vi "Keithley 2600 Series Merge NEW.vi"() -> ()   [LabVIEW 2017]
doc: "This example shows how to create, run a script and query the script output data."
uses:
  <vilib>/Utility/file.llb/Write Delimited Spreadsheet (DBL).vi
  <instrlib>/Keithley 2600 Series/Keithley 2600 Series.lvlib
panel:
  out "Sweep":i32
  in  "Yes":bool
  out "First Sweep 2":bool
  in  "No":bool
  out "Graph 2":cluster{"Y":dbl[], "Y":dbl[]}[](graph)
  out "output array":string[][](array[string])
  out "Seconds":i32
  out "Minutes":i32
  out "Hours":i32
  in  "Stop Button":bool
  in  "Number of Sweeps":dbl=10.0 min=1.0 max=1000.0 step=1.0
  in  "Aperture State (Channel B)":u16(ring) items=["Always OFF", "Always ON", "ON During Sweep OFF Otherwise", "OFF During Sweep ON Otherwise"]
  in  "Inter Sweep Delay(s)":dbl=0.1 min=0.1 max=3600.0
  out "Working Folder":path
  in  "Folder Name":string="Raw Measurement"
  in  "Sweep Setting (Channel A)":T1={"Start Voltage(V)"=0.0, "Stop Voltage(V)"=0.0, "Number of Points"=10.0, "Settling Time(s)"=0.1, "Current Limit(A)"=0.1} {"Current Limit(A)" min=0.1 max=1.5; "Settling Time(s)" min=0.1 max=60.0; "Number of Points" min=10.0 max=10000.0 step=1.0; "Stop Voltage(V)" min=0.0 max=200.0; "Start Voltage(V)" min=0.0 max=200.0}
  in  "USB COM Port":refnum<visa-resource-name>
  # "Time Remaining"
  # ":"
  # ":"
  # "2634B can output up to 20.2 V at 1.5 A,\n or 202 V at 100 mA current limit."
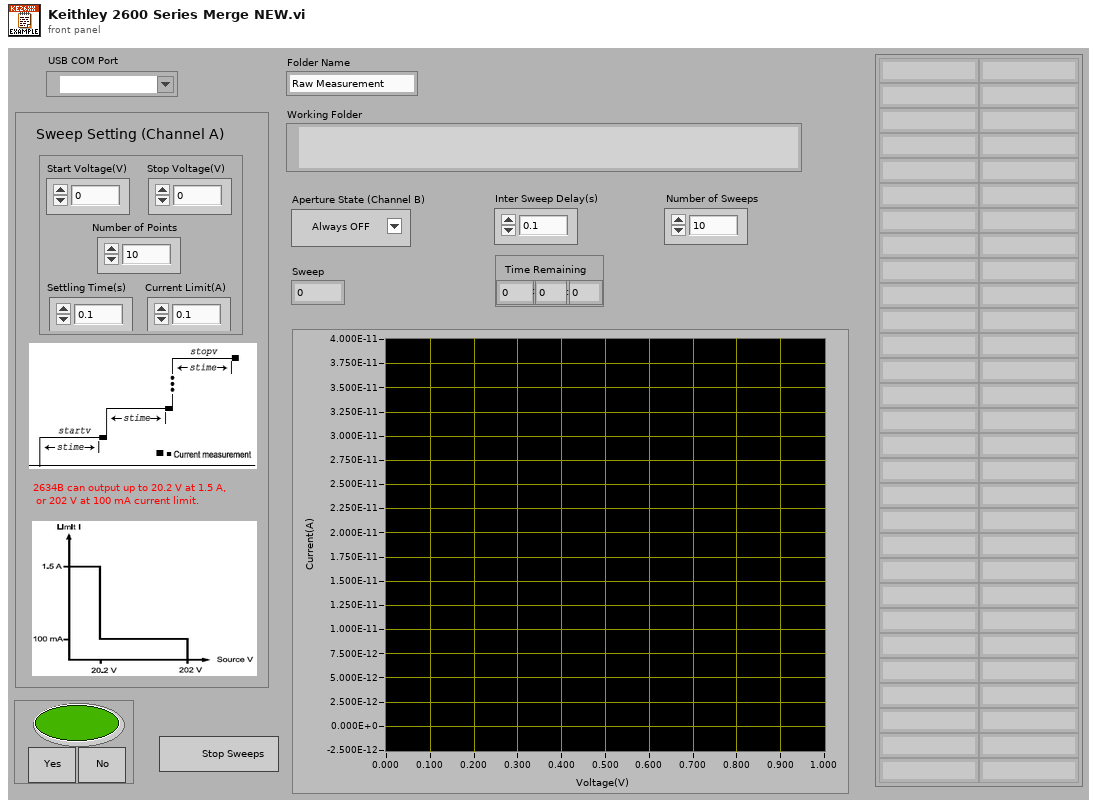
[diagram p1: front panel]
types:
  T1 = cluster{"Start Voltage(V)":dbl, "Stop Voltage(V)":dbl, "Number of Points":dbl, "Settling Time(s)":dbl, "Current Limit(A)":dbl}
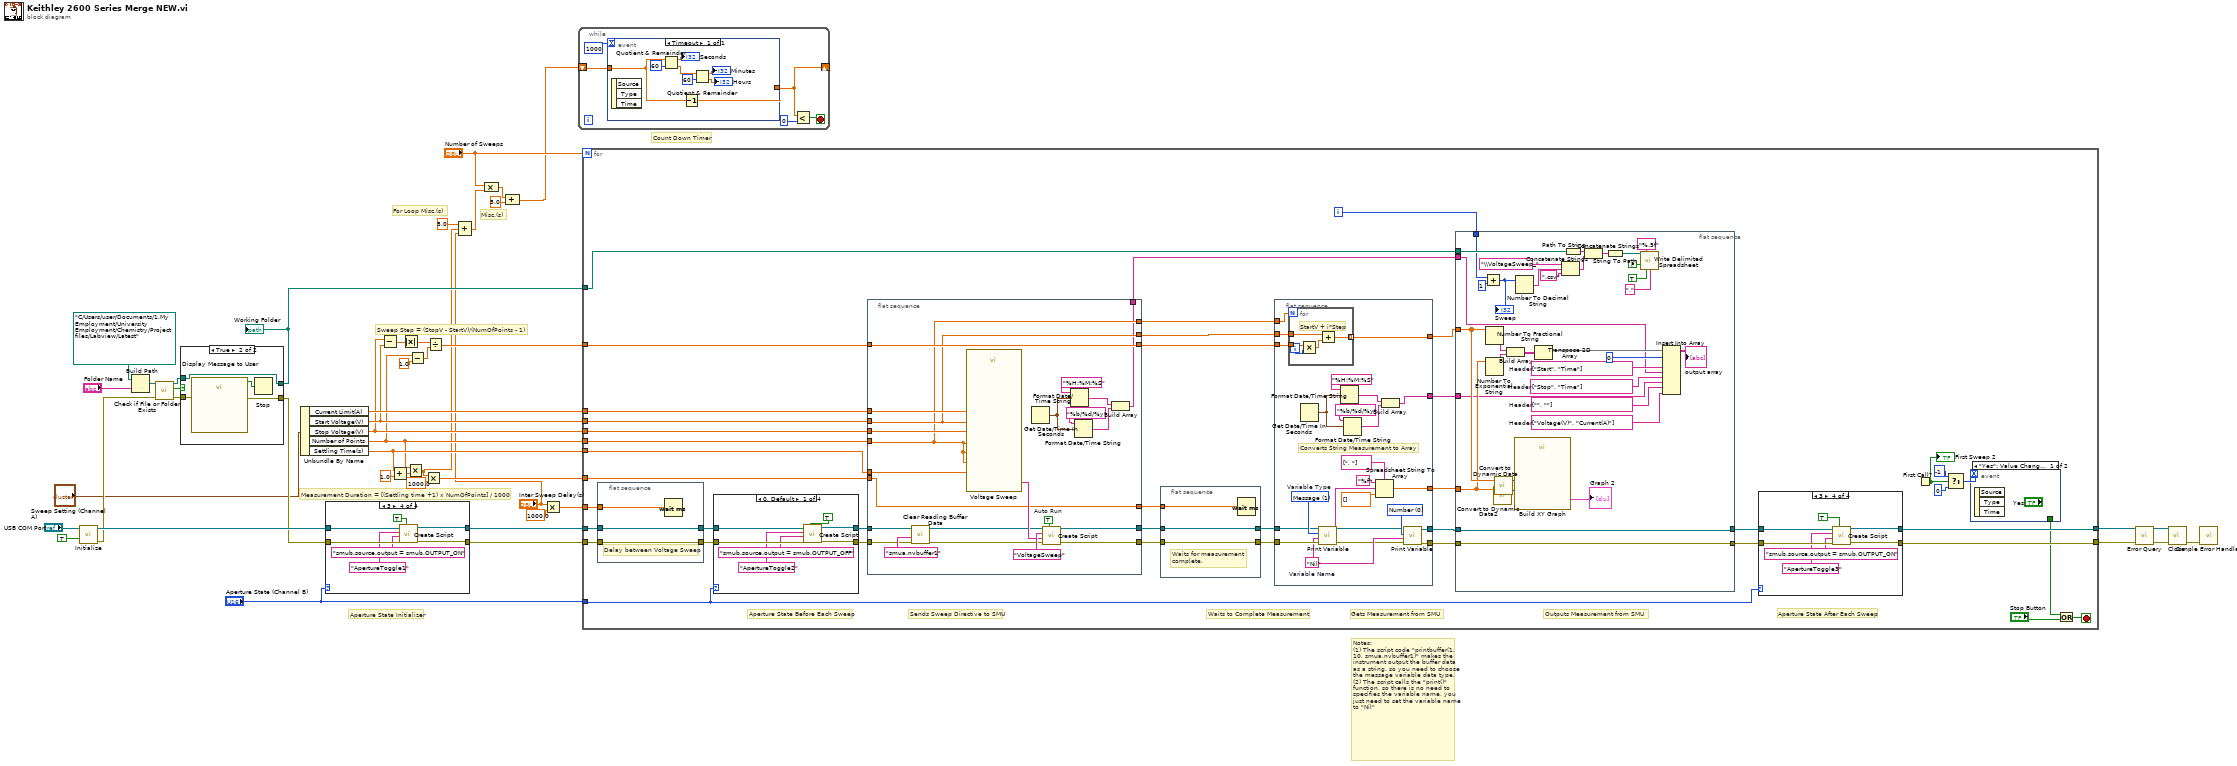
[diagram p0: block diagram]
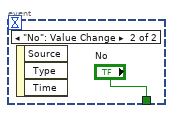
[diagram p2: hidden frame]
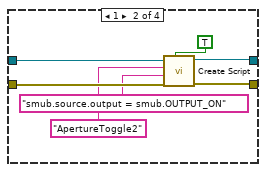
[diagram p3: hidden frame]
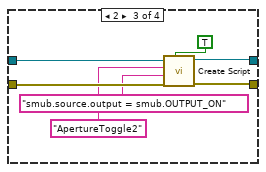
[diagram p4: hidden frame]
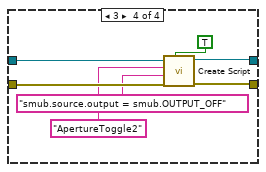
[diagram p5: hidden frame]
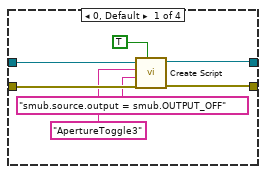
[diagram p6: hidden frame]
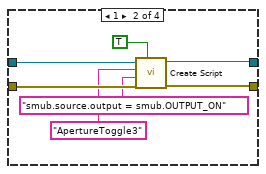
[diagram p7: hidden frame]
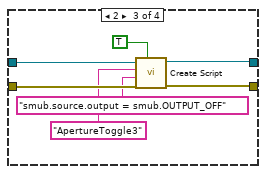
[diagram p8: hidden frame]
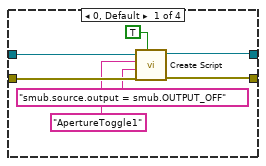
[diagram p9: hidden frame]
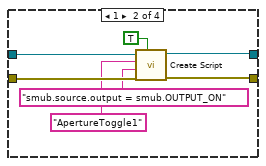
[diagram p10: hidden frame]
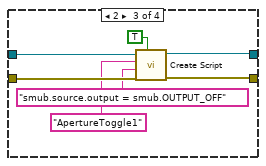
[diagram p11: hidden frame]
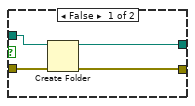
[diagram p12: hidden frame]
diagram:
  # "Count Down Timer"
  # "Misc.(s)"
  # "For Loop Misc.(s)"
  # "Sweep Step = (StopV - StartV)/(NumOfPoints - 1)"
  # "Measurement Duration = [(Settling time +1) x NumOfPoints] / 1000"
  # "Aperture State Initializer"
  # "Notes: \n(1) The script code \"printbuffer(1, 10, smua.nvbuffer1)\" makes the instrument output the buffer data as a string, so you need to choose the message variable data type.\n(2) The script calls the \"print()\" function, so there is no need to specifies the variable name, you just need to set the variable name to \"Nil\""
  n1 = call <instrlib>:"Initialize.vi"("Reset (True)"=TRUE, "VISA resource name"="USB COM Port") -> ("error out"=w28:errorcluster, "VISA resource name out"=w29:refnum<visa-resource-name>)  [unwired: 8 in]
  n2 = Build Path(base path=path "C:/Users/user/Documents/1.My Employment/University Employment/Chemistry/Project files/Labview/Latest" ("Working Directory"), name or relative path="Folder Name") -> (appended path=w38:path)
  n3 = call <vilib>:"Check if File or Folder Exists.vi"("error in (no error)"=w28, "path"=w38) -> ("error out"=w35:errorcluster, "file or folder exists?"=w37:bool, "dup path"=w36:path)  [unwired: 7 in]
  n4 = case shown="True" w37 {
    tunnel: [w48 w51] -> w34
    tunnel: w36 -> [w49 w51]
    tunnel: w35 -> [w47 w53]
    tunnel: [w46 w50] -> w27
    frame False {
      n5 = Create Folder(path (use dialog)=w49, error in=w47) -> (created path=w48:path, error out=w46:errorcluster)  [unwired: 1 in, 1 out]
    }
    frame True {
      n6 = call "Display Message to User"("error in (no error)"=w53) -> ("error out"=w50:errorcluster, "OK"=w52:bool)  [unwired: 9 in]
      n7 = Stop(stop? (T)=w52) -> ()
    }
  }
  "Working Folder" <- w34
  n8 = Unbundle By Name("Sweep Setting (Channel A)") -> ("Current Limit(A)"=w24:dbl, "Start Voltage(V)"=w13:dbl, "Stop Voltage(V)"=w12:dbl, "Number of Points"=w11:dbl, "Settling Time(s)"=w22:dbl)
  n9 = case shown="3" "Aperture State (Channel B)" {
    tunnel: w29 -> [w60 w67 w74 w81]
    tunnel: w27 -> [w57 w64 w71 w78]
    tunnel: [w59 w66 w73 w80] -> w31
    tunnel: [w58 w65 w72 w79] -> w30
    frame 0, Default {
      n10 = call <instrlib>:"Create Script.vi"("Auto Run (F: Disable)"=TRUE, "error in (no error)"=w57, "Source Code"="smub.source.output = smub.OUTPUT_OFF", "Script Variable"="ApertureToggle1", "VISA resource name"=w60) -> ("error out"=w58:errorcluster, "VISA resource name out"=w59:refnum<visa-resource-name>)  [unwired: 5 in]
    }
    frame 1 {
      n11 = call <instrlib>:"Create Script.vi"("Auto Run (F: Disable)"=TRUE, "error in (no error)"=w64, "Source Code"="smub.source.output = smub.OUTPUT_ON", "Script Variable"="ApertureToggle1", "VISA resource name"=w67) -> ("error out"=w65:errorcluster, "VISA resource name out"=w66:refnum<visa-resource-name>)  [unwired: 5 in]
    }
    frame 2 {
      n12 = call <instrlib>:"Create Script.vi"("Auto Run (F: Disable)"=TRUE, "error in (no error)"=w71, "Source Code"="smub.source.output = smub.OUTPUT_OFF", "Script Variable"="ApertureToggle1", "VISA resource name"=w74) -> ("error out"=w72:errorcluster, "VISA resource name out"=w73:refnum<visa-resource-name>)  [unwired: 5 in]
    }
    frame 3 {
      n13 = call <instrlib>:"Create Script.vi"("Auto Run (F: Disable)"=TRUE, "error in (no error)"=w78, "Source Code"="smub.source.output = smub.OUTPUT_ON", "Script Variable"="ApertureToggle1", "VISA resource name"=w81) -> ("error out"=w79:errorcluster, "VISA resource name out"=w80:refnum<visa-resource-name>)  [unwired: 5 in]
    }
  }
  n14 = Subtract(x=w12, y=w13) -> (x-y=w17:dbl)
  n15 = Add(x=w22, y=1.0) -> (x+y=w21:dbl)
  n16 = Absolute Value(x=w17) -> (abs(x)=w18:dbl)
  n17 = Multiply(x=w11, y=w21) -> (x*y=w4:dbl)
  n18 = Subtract(x=w11, y=1.0) -> (x-y=w16:dbl)
  n19 = Multiply(x=w4, y=1000.0) -> (x*y=w3:dbl)
  n20 = Divide(x=w18, y=w16) -> (x/y=w14:dbl)
  n21 = Compound Arithmetic op=ADD(5.0 ("value"), w4, "Inter Sweep Delay(s)") -> (w8:dbl)
  n22 = Compound Arithmetic op=MULTIPLY("Number of Sweeps", w8) -> (w7:dbl)
  n23 = Compound Arithmetic op=ADD(w7, 5.0 ("value")) -> (w5:dbl)
  n24 = Multiply(x="Inter Sweep Delay(s)", y=1000.0) -> (x*y=w1:dbl)
  n25 = while {
    shift-right: [w83] -> _
    shift-left: w5 -> [w85]
    stop <- w84 stop-if-true
    n26 = event shown="[0] Timeout" {
      selector: _ -> [_]
      dyn-events: _ -> [_]
      timeout: 1000 -> [_]
      tunnel: w85 -> [w92]
      tunnel: [w94] -> w83
      event Timeout {
        n27 = event-data() -> ()  [unwired: 1 in, 3 out]
        n28 = Quotient & Remainder(x=w92, y=60) -> (x-y*floor(x/y)=→"Seconds":dbl, floor(x/y)=w88:dbl)
        n29 = Decrement(x=w92) -> (x-1=w94:dbl)
        n30 = Quotient & Remainder(x=w88, y=60) -> (x-y*floor(x/y)=→"Minutes":dbl, floor(x/y)=→"Hours":dbl)
      }
    }
    n31 = Less?(x=w83, y=0) -> (x < y?=w84:bool)
  }
  n32 = for {
    N: "Number of Sweeps" -> [_]
    tunnel: w34 -> [w107]
    tunnel: "Aperture State (Channel B)" -> [w126]
    tunnel: w31 -> [w130]
    tunnel: [w104] -> w33
    tunnel: w30 -> [w129]
    tunnel: [w103] -> w32
    tunnel: w24 -> [w125]
    tunnel: w13 -> [w119]
    tunnel: w12 -> [w118]
    tunnel: w11 -> [w120]
    tunnel: w22 -> [w124]
    tunnel: w3 -> [w123]
    tunnel: w1 -> [w121]
    tunnel: w14 -> [w117]
    i -> [w98]
    stop <- w97 stop-if-true
    # "Aperture State Before Each Sweep"
    # "Aperture State After Each Sweep"
    # "Sends Sweep Directive to SMU"
    # "Waits to Complete Measurement"
    # "Outputs Measurement from SMU"
    # "Gets Measurement from SMU"
    n33 = flat-sequence {
      tunnel: w130 -> [w174]
      tunnel: w129 -> [w173]
      tunnel: [w174] -> w128
      tunnel: [w173] -> w127
      tunnel: w121 -> [w172]
      frame #0 {
        # "Delay between Voltage Sweep"
        n34 = Wait (ms)(milliseconds to wait=w172) -> ()  [unwired: 1 out]
      }
    }
    n35 = case shown="0, Default" w126 {
      tunnel: w128 -> [w181 w188 w195 w202]
      tunnel: w127 -> [w178 w185 w192 w199]
      tunnel: [w180 w187 w194 w201] -> w132
      tunnel: [w179 w186 w193 w200] -> w131
      frame 0, Default {
        n36 = call <instrlib>:"Create Script.vi"("Auto Run (F: Disable)"=TRUE, "error in (no error)"=w178, "Source Code"="smub.source.output = smub.OUTPUT_OFF", "Script Variable"="ApertureToggle2", "VISA resource name"=w181) -> ("error out"=w179:errorcluster, "VISA resource name out"=w180:refnum<visa-resource-name>)  [unwired: 5 in]
      }
      frame 1 {
        n37 = call <instrlib>:"Create Script.vi"("Auto Run (F: Disable)"=TRUE, "error in (no error)"=w185, "Source Code"="smub.source.output = smub.OUTPUT_ON", "Script Variable"="ApertureToggle2", "VISA resource name"=w188) -> ("error out"=w186:errorcluster, "VISA resource name out"=w187:refnum<visa-resource-name>)  [unwired: 5 in]
      }
      frame 2 {
        n38 = call <instrlib>:"Create Script.vi"("Auto Run (F: Disable)"=TRUE, "error in (no error)"=w192, "Source Code"="smub.source.output = smub.OUTPUT_ON", "Script Variable"="ApertureToggle2", "VISA resource name"=w195) -> ("error out"=w193:errorcluster, "VISA resource name out"=w194:refnum<visa-resource-name>)  [unwired: 5 in]
      }
      frame 3 {
        n39 = call <instrlib>:"Create Script.vi"("Auto Run (F: Disable)"=TRUE, "error in (no error)"=w199, "Source Code"="smub.source.output = smub.OUTPUT_OFF", "Script Variable"="ApertureToggle2", "VISA resource name"=w202) -> ("error out"=w200:errorcluster, "VISA resource name out"=w201:refnum<visa-resource-name>)  [unwired: 5 in]
      }
    }
    n40 = flat-sequence {
      tunnel: [w275] -> w134
      tunnel: [w276] -> w133
      tunnel: w132 -> [w282]
      tunnel: w131 -> [w280]
      tunnel: w125 -> [w272]
      tunnel: w119 -> [w267]
      tunnel: w118 -> [w271]
      tunnel: w120 -> [w266]
      tunnel: w124 -> [w270]
      tunnel: w123 -> [w269]
      tunnel: [w269] -> w122
      tunnel: w117 -> [w268]
      tunnel: [w268] -> w116
      tunnel: [w267] -> w115
      tunnel: [w266] -> w114
      tunnel: [w260] -> w108
      frame #0 {
        w278 = TRUE  # Auto Run
        n41 = call <instrlib>:"Clear Reading Buffer Data.vi"("error in (no error)"=w280, "Reading Buffer (smua.nvbuffer1)"="smua.nvbuffer1", "VISA resource name"=w282) -> ("error out"=w273:errorcluster, "VISA resource name out"=w274:refnum<visa-resource-name>)  [unwired: 7 in]
        n42 = call "Voltage Sweep"("StopV"=w271, "LevelNumber1"=w266, "CurrentLimit"=w272, "SettlingTime"=w270, "StartV"=w267, "LevelNumber0"=w266, "LevelNumber2"=w266) -> ("Result"=w277:string)  [unwired: 7 in, 1 out]
        n43 = Get Date/Time In Seconds() -> (seconds since 1Jan1904=w261:timestamp)
        n44 = call <instrlib>:"Create Script.vi"("Auto Run (F: Disable)"=w278, "error in (no error)"=w273, "Source Code"=w277, "Script Variable"="VoltageSweep", "VISA resource name"=w274) -> ("error out"=w276:errorcluster, "VISA resource name out"=w275:refnum<visa-resource-name>)  [unwired: 5 in]
        n45 = Format Date/Time String(time format string (%c)="%H:%M:%S", seconds (now)=w261) -> (date/time string=w264:string)  [unwired: 1 out]
        n46 = Format Date/Time String(time format string (%c)="%b/%d/%y", seconds (now)=w261) -> (date/time string=w262:string)  [unwired: 1 out]
        n47 = Build Array(w264, w262) -> (w260:string[])
      }
    }
    n48 = flat-sequence {
      tunnel: w134 -> [w284]
      tunnel: w133 -> [w285]
      tunnel: [w285] -> w135
      tunnel: [w284] -> w136
      tunnel: w122 -> [w283]
      frame #0 {
        # "Waits for measurement complete."
        n49 = Wait (ms)(milliseconds to wait=w283) -> ()  [unwired: 1 out]
      }
    }
    n50 = flat-sequence {
      tunnel: w136 -> [w253]
      tunnel: w135 -> [w252]
      tunnel: [w247] -> w112
      tunnel: [w242] -> w110
      tunnel: w116 -> [w241]
      tunnel: w115 -> [w240]
      tunnel: w114 -> [w239]
      tunnel: [w238] -> w113
      tunnel: [w237] -> w111
      tunnel: [w231] -> w109
      frame #0 {
        w244 = 0 items=["Number", "Message"] ("Variable Type (0: Number)")
        w254 = 1 items=["Number", "Message"]  # Variable Type
        w246 = "Nil"  # Variable Name
        # "Converts String Measurement to Array"
        n51 = for {
          N: w239 -> [_]
          tunnel: w241 -> [w258]
          tunnel: [w256] -> w238 mode=indexing
          tunnel: w240 -> [w255]
          i -> [w259]
          # "StartV + i*Step"
          n52 = Multiply(x=w258, y=w259) -> (x*y=w257:dbl)
          n53 = Add(x=w255, y=w257) -> (x+y=w256:dbl)
        }
        n54 = Get Date/Time In Seconds() -> (seconds since 1Jan1904=w232:timestamp)
        n55 = call <instrlib>:"Print Variable.vi"("error in (no error)"=w252, "Variable Name"=w246, "Variable Type (0: Number)"=w254, "VISA resource name"=w253) -> ("error out"=w245:errorcluster, "Message"=w251:string, "VISA resource name out"=w243:refnum<visa-resource-name>)  [unwired: 4 in, 1 out]
        n56 = Format Date/Time String(time format string (%c)="%H:%M:%S", seconds (now)=w232) -> (date/time string=w235:string)  [unwired: 1 out]
        n57 = Format Date/Time String(time format string (%c)="%b/%d/%y", seconds (now)=w232) -> (date/time string=w233:string)  [unwired: 1 out]
        n58 = Spreadsheet String To Array(delimiter (Tab)=string[] [", "], format string="%f", spreadsheet string=w251, array type (2D Dbl)=dbl[] []) -> (array=w247:dbl[])
        n59 = Build Array(w235, w233) -> (w231:string[])
        n60 = call <instrlib>:"Print Variable.vi"("error in (no error)"=w245, "Variable Name"=w246, "Variable Type (0: Number)"=w244, "VISA resource name"=w243) -> ("error out"=w242:errorcluster, "VISA resource name out"=w237:refnum<visa-resource-name>)  [unwired: 4 in, 2 out]
      }
    }
    n61 = flat-sequence {
      tunnel: w112 -> [w150]
      tunnel: w107 -> [w155]
      tunnel: w113 -> [w151]
      tunnel: w110 -> [w157]
      tunnel: [w157] -> w105
      tunnel: [w156] -> w106
      tunnel: w111 -> [w156]
      tunnel: w108 -> [w144]
      tunnel: w109 -> [w143]
      tunnel: w98 -> [w138]
      frame #0 {
        w140 = string[] ["Voltage(V)", "Current(A)"]  # Header
        w141 = string[] ["", ""]  # Header
        w142 = string[] ["Stop", "Time"]  # Header
        w146 = string[] ["Start", "Time"]  # Header
        n62 = Add(x=w138, y=1 ("x")) -> (x+y=w158:i32)
        "Sweep" <- w158
        n63 = Number To Fractional String(number=w151) -> (F-format string=w153:string[])  [unwired: 3 in]
        n64 = Number To Exponential String(number=w150) -> (E-format string=w152:string[])  [unwired: 3 in]
        n65 = call "Convert to Dynamic Data2"("Array"=w150) -> ("Dynamic Data Type"=w170:dynamicdata)  [unwired: 3 in]
        n66 = call "Convert to Dynamic Data"("Array"=w151) -> ("Dynamic Data Type"=w171:dynamicdata)  [unwired: 3 in]
        n67 = Build Array(w153, w152) -> (w154:string[][])
        n68 = call "Build XY Graph"("Y Input"=w170, "X Input"=w171) -> ("XY Graph"=→"Graph 2":cluster{"X":dbl[], "Y":dbl[]}[])  [unwired: 8 in, 1 out]
        n69 = Number To Decimal String(number=w158) -> (decimal integer string=w159:string)  [unwired: 1 in]
        n70 = Transpose 2D Array(2D array=w154) -> (transposed array=w148:string[][])
        n71 = Concatenate Strings("\\VoltageSweep_" ("string"), w159, ".csv" ("string")) -> (w162:string)
        n72 = Path To String(path=w155) -> (string=w168:string)
        n73 = Concatenate Strings(w168, w162) -> (w167:string)
        n74 = String To Path(string=w167) -> (path=w166:path)
        n75 = call-poly <vilib>:"Write Delimited Spreadsheet.vi"("file path (dialog if empty)"=w166, "format (%.3f)"="%.5f", "append to file? (new file:F)"=FALSE, "transpose? (no:F)"=TRUE, "delimiter (\\t)"="," ("delimiter (\\t)")) -> ()  [unwired: 9 in, 2 out]
        n76 = Insert Into Array(array=w148, index (row)=0, new element #1=w146, new element #2=w144, new element #3=w142, new element #4=w143, new element #5=w141, new element #6=w140) -> (→"output array":string[][])  [unwired: 1 in]
      }
    }
    n77 = case shown="3" w126 {
      tunnel: w106 -> [w209 w216 w223 w230]
      tunnel: w105 -> [w206 w213 w220 w227]
      tunnel: [w208 w215 w222 w229] -> w104
      tunnel: [w207 w214 w221 w228] -> w103
      frame 0, Default {
        n78 = call <instrlib>:"Create Script.vi"("Auto Run (F: Disable)"=TRUE, "error in (no error)"=w206, "Source Code"="smub.source.output = smub.OUTPUT_OFF", "Script Variable"="ApertureToggle3", "VISA resource name"=w209) -> ("error out"=w207:errorcluster, "VISA resource name out"=w208:refnum<visa-resource-name>)  [unwired: 5 in]
      }
      frame 1 {
        n79 = call <instrlib>:"Create Script.vi"("Auto Run (F: Disable)"=TRUE, "error in (no error)"=w213, "Source Code"="smub.source.output = smub.OUTPUT_ON", "Script Variable"="ApertureToggle3", "VISA resource name"=w216) -> ("error out"=w214:errorcluster, "VISA resource name out"=w215:refnum<visa-resource-name>)  [unwired: 5 in]
      }
      frame 2 {
        n80 = call <instrlib>:"Create Script.vi"("Auto Run (F: Disable)"=TRUE, "error in (no error)"=w220, "Source Code"="smub.source.output = smub.OUTPUT_OFF", "Script Variable"="ApertureToggle3", "VISA resource name"=w223) -> ("error out"=w221:errorcluster, "VISA resource name out"=w222:refnum<visa-resource-name>)  [unwired: 5 in]
      }
      frame 3 {
        n81 = call <instrlib>:"Create Script.vi"("Auto Run (F: Disable)"=TRUE, "error in (no error)"=w227, "Source Code"="smub.source.output = smub.OUTPUT_ON", "Script Variable"="ApertureToggle3", "VISA resource name"=w230) -> ("error out"=w228:errorcluster, "VISA resource name out"=w229:refnum<visa-resource-name>)  [unwired: 5 in]
      }
    }
    n82 = First Call?() -> (First Call?: T/F=w99:bool)
    "First Sweep 2" <- w99
    n83 = Select(t=-1, s=w99, f=0) -> (s? t:f=w100:i32)
    n84 = event shown="[0] \"Yes\": Value Change;  Timeout" {
      selector: _ -> [_ _]
      dyn-events: _ -> [_ _]
      timeout: w100 -> [_ _]
      tunnel: [_ "No"] -> w95
      event "Yes": Value Change; Timeout {
        n85 = event-data() -> ()  [unwired: 1 in, 3 out]
      }
      event "No": Value Change {
        n86 = event-data() -> ()  [unwired: 1 in, 3 out]
      }
    }
    n87 = Or(x=w95, y="Stop Button") -> (x .or. y?=w97:bool)
  }
  n88 = call <instrlib>:"Error Query.vi"("error in (no error)"=w32, "VISA resource name"=w33) -> ("error out"=w43:errorcluster, "VISA resource name out"=w44:refnum<visa-resource-name>)  [unwired: 6 in, 2 out]
  n89 = call <instrlib>:"Close.vi"("error in (no error)"=w43, "VISA resource name"=w44) -> ("error out"=w45:errorcluster)  [unwired: 9 in]
  n90 = call <vilib>:"Simple Error Handler.vi"("error in (no error)"=w45) -> ()  [unwired: 4 in, 5 out]
